vi "handle_CAN_error.vi"(11 "error in (no error)":errorcluster) -> (1 "stop":bool, 3 "error out":errorcluster)   [LabVIEW 2020]
uses:
  <vilib>/ErrorRing/Error Ring.xnode
  <vilib>/Utility/SystemLogging/NI_SystemLogging.lvlib
panel:
  in  "retry delay (ms)":u32=500
  in  "# of tries":i32=3
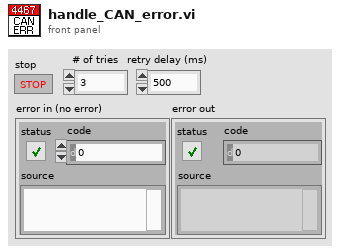
[diagram p1: front panel]
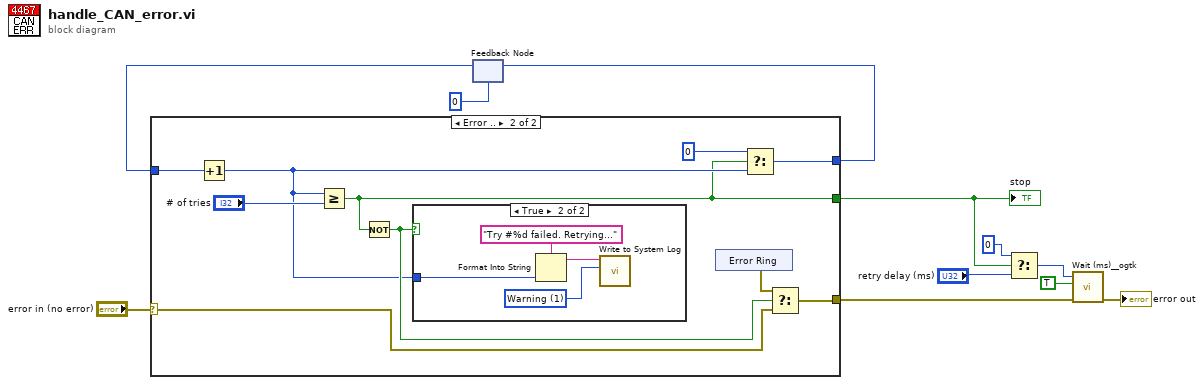
[diagram p0: block diagram]
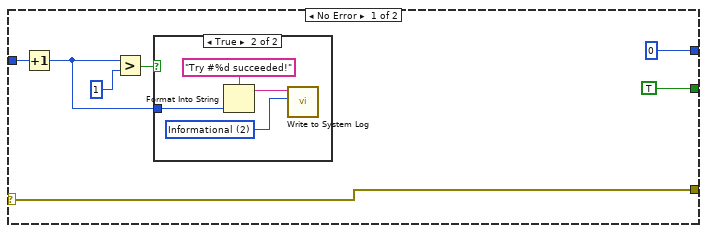
[diagram p2: hidden frame]
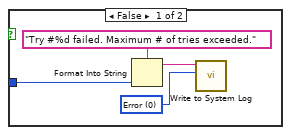
[diagram p4: hidden frame]
diagram:
  n1 = feedback #1(0) -> (w9:i32)
  n2 = case shown="Error .." "error in (no error)" {
    selector: "error in (no error)" -> [w16 w23]
    tunnel: w9 -> [w15 w32]
    tunnel: [0 w24] -> w8
    tunnel: [TRUE ("stop") w26] -> w6
    tunnel: [w16 w30] -> w4
    frame No Error {
      n3 = Increment(x=w15) -> (x+1=w13:i32)
      n4 = Greater?(x=w13, y=1) -> (0:w12:bool)
      n5 = case shown="True" w12 {
        tunnel: w13 -> [_ w21]
        frame False {
        }
        frame True {
          w20 = 2 items=["Error", "Warning", "Informational"] ("severity")
          n6 = Format Into String(format string="Try #%d succeeded!" ("message"), w21) -> (resulting string=w19:string)  [unwired: 2 in, 1 out]
          n7 = call <vilib>:"Write to System Log.vi"("severity"=w20, "message"=w19) -> ()  [unwired: 9 in, 1 out]
        }
      }
    }
    frame Error {
      n8 = Increment(x=w32) -> (x+1=w27:i32)
      n9 = Greater Or Equal?(x=w27, y="# of tries") -> (x >= y?=w26:bool)
      n10 = Not(x=w26) -> (.not. x?=w28:bool)
      n11 = case shown="True" w28 {
        tunnel: w27 -> [w33 w39]
        frame False {
          w35 = 0 items=["Error", "Warning", "Informational"] ("severity")
          n12 = Format Into String(format string="Try #%d failed. Maximum # of tries exceeded." ("message"), w33) -> (resulting string=w36:string)  [unwired: 2 in, 1 out]
          n13 = call <vilib>:"Write to System Log.vi"("severity"=w35, "message"=w36) -> ()  [unwired: 9 in, 1 out]
        }
        frame True {
          w38 = 1 items=["Error", "Warning", "Informational"] ("severity")
          n14 = Format Into String(format string="Try #%d failed. Retrying..." ("message"), w39) -> (resulting string=w37:string)  [unwired: 2 in, 1 out]
          n15 = call <vilib>:"Write to System Log.vi"("severity"=w38, "message"=w37) -> ()  [unwired: 9 in, 1 out]
        }
      }
      n16 = xnode "Error Ring"() -> ("error out"=w29:errorcluster)
      n17 = Select(t=0, s=w26, f=w27) -> (s? t:f=w24:i32)
      n18 = Select(t=w29, s=w28, f=w23) -> (s? t:f=w30:errorcluster)
    }
  }
  "stop" <- w6
  n19 = feedback-in #1(w8) -> ()
  n20 = Select(t=u32 0, s=w6, f="retry delay (ms)") -> (s? t:f=w1:u32)
  n21 = call "Wait (ms)__ogtk.vi"("error in (no error)"=w4, "Wait on Error (FALSE)"=TRUE, "milliseconds to wait"=w1) -> ("error out"=→"error out":errorcluster)  [unwired: 7 in, 1 out]
